vi "Configure SPI.vi"(8 "error in (no error)":errorcluster, 10 "SPI Message Byte":u8[](array[numeric]) format="%.0x", 11 "VISA resource name":refnum<visa-resource-name>) -> (0 "error out":errorcluster, 2 "SPI Message Output":string, 3 "VISA resource name out":refnum<visa-resource-name>)   [LabVIEW 2021, in "Ocean Optics 2000 4000.lvlib"]
doc: "Configures the SPI Input/Output on the SPI bus for interfacing with attached peripherals. Time to complete the command is determined by the amount of data transfer and response time of the peripheral. SPI bus runs at ~25KHz clock."
uses:
  <instrlib>/Ocean Optics 2000 4000/Ocean Optics 2000 4000.lvlib
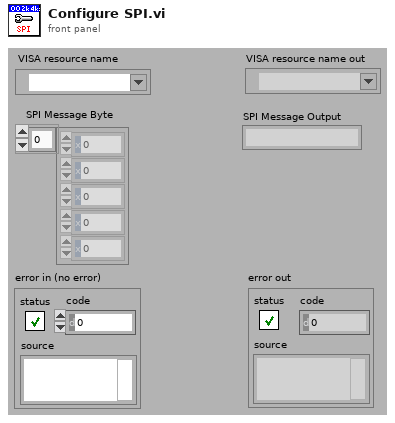
[diagram p1: front panel]
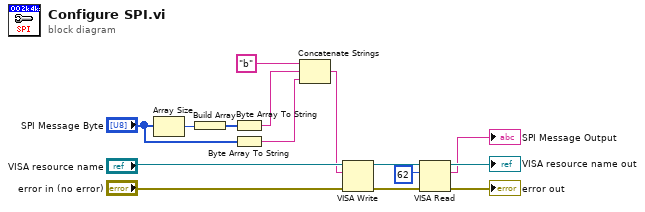
[diagram p0: block diagram]
diagram:
  n1 = Array Size(array="SPI Message Byte") -> (size(s)=w11:i32)
  n2 = Build Array(w11) -> (w12:i32[])
  n3 = Byte Array To String(unsigned byte array=w12) -> (string=w10:string)
  n4 = Byte Array To String(unsigned byte array="SPI Message Byte") -> (string=w8:string)
  n5 = Concatenate Strings("b" ("string"), w10, w8) -> (w7:string)
  n6 = VISA Write(VISA resource name="VISA resource name", write buffer=w7, error in (no error)="error in (no error)") -> (VISA resource name out=w6:refnum<visa-resource-name>, error out=w3:errorcluster)  [unwired: 1 out]
  n7 = VISA Read(VISA resource name=w6, byte count=u32 62, error in (no error)=w3) -> (VISA resource name out=→"VISA resource name out":refnum<visa-resource-name>, read buffer=→"SPI Message Output":string, error out=→"error out":errorcluster)  [unwired: 1 out]
